vi "LINC Read Packet Names.vi"(8 "error in (no error)":errorcluster, 10 "type":enum16{"CMD", "TLM"}(ring), 11 "LINC session":refnum<class "LINC.lvclass">) -> (0 "error out":errorcluster, 1 "packet descriptions":string[](array[string]), 2 "packet names":string[](array[string]), 3 "dup LINC session":refnum<class "LINC.lvclass">, 4 "hazardous":bool[](array[boolean]))   [LabVIEW 2018, in "STEPkgDriver_LINC.lvlib" / "LINC.lvclass"]
doc: "Reads the available packet names, descriptions, and hazardous information for a LINC session."
uses:
  LINC.lvclass
  LINC Global Mode.ctl
  STEPkgDriver_LINC.lvlib
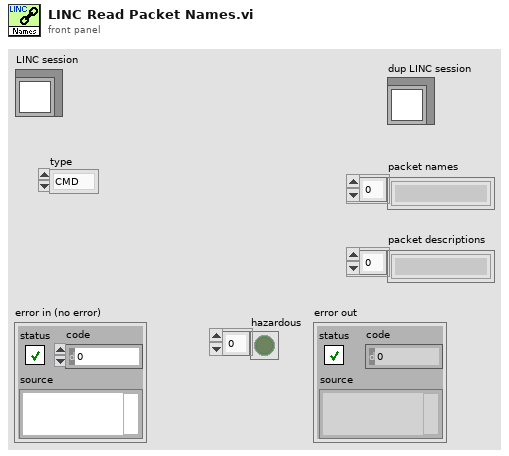
[diagram p1: front panel]
types:
  T1 = typedef "STEPkgDriver_LINC.lvlib/LINC Global Mode.ctl" = enum16{"INIT", "CLEAR", "ADD_PKT_HDR", "ADD_PKT", "GET_PKT_NAMES", "GET_PKT_DESC", "GET_PKT_HDR", "GET_PKT", "SET_PKT", "SET_DATA", "SIM_EN", "SIM_DS"}
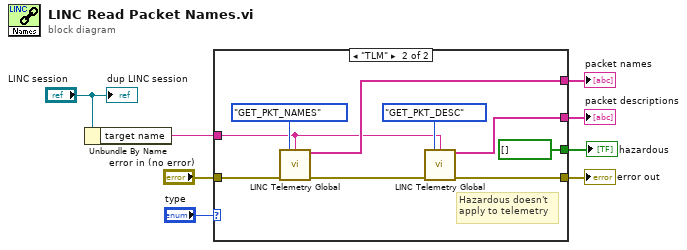
[diagram p0: block diagram]
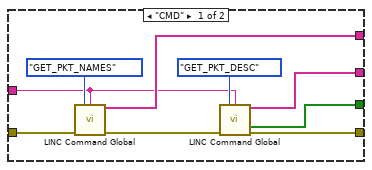
[diagram p2: hidden frame]
diagram:
  n1 = Unbundle By Name("LINC session") -> ("target name"=w6:string)
  n2 = case shown="\"TLM\"" "type" {
    tunnel: "error in (no error)" -> [w16 w25]
    tunnel: [w12 w21] -> w7
    tunnel: w6 -> [w11 w20]
    tunnel: [w15 w24] -> w4
    tunnel: [w10 w19] -> w2
    tunnel: [w9 bool[] [] ("hazardous out")] -> w1
    frame "CMD" {
      n3 = call "LINC Command Global.vi"("mode"=LINC_Global_Mode."GET_PKT_NAMES", "target name"=w11, "error in (no error)"=w16) -> ("values out"=w15:string[], "error out"=w13:errorcluster)  [unwired: 8 in, 3 out]
      n4 = call "LINC Command Global.vi"("mode"=LINC_Global_Mode."GET_PKT_DESC", "target name"=w11, "error in (no error)"=w13) -> ("values out"=w10:string[], "hazardous out"=w9:bool[], "error out"=w12:errorcluster)  [unwired: 8 in, 2 out]
    }
    frame "TLM" {
      # "Hazardous doesn't\napply to telemetry"
      n5 = call "LINC Telemetry Global.vi"("mode"=LINC_Global_Mode."GET_PKT_NAMES", "target name"=w20, "error in (no error)"=w25) -> ("values out"=w24:string[], "error out"=w22:errorcluster)  [unwired: 8 in, 3 out]
      n6 = call "LINC Telemetry Global.vi"("mode"=LINC_Global_Mode."GET_PKT_DESC", "target name"=w20, "error in (no error)"=w22) -> ("values out"=w19:string[], "error out"=w21:errorcluster)  [unwired: 8 in, 3 out]
    }
  }
  "error out" <- w7
  "packet names" <- w4
  "packet descriptions" <- w2
  "hazardous" <- w1
  "dup LINC session" <- "LINC session"
